vi "PromVIEW_GlobalOnCommand.vi"(10 "Command ID":string, 11 "Item Ref":T1) -> ()   [LabVIEW 2020]
uses:
  <resource>/Framework/Providers/API/ItemRef.ctl
panel:
  out "error out":errorcluster
  in  "error in":errorcluster
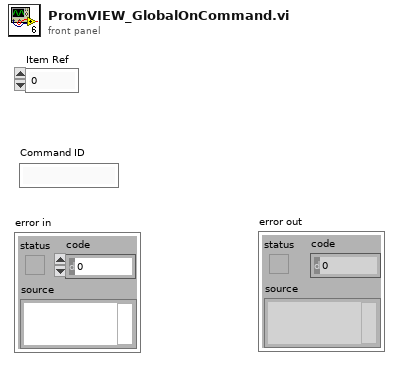
[diagram p1: front panel]
types:
  T1 = typedef "ItemRef.ctl" = u64
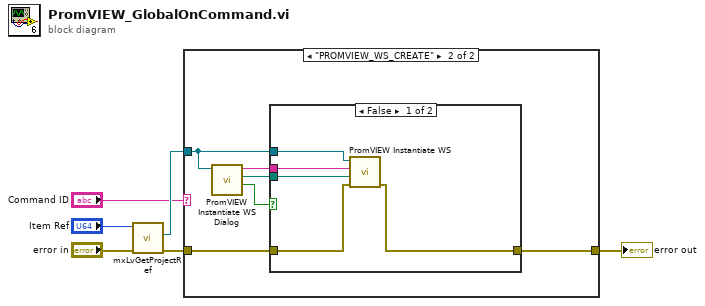
[diagram p0: block diagram]
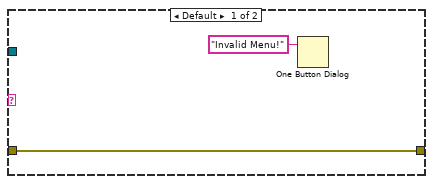
[diagram p2: hidden frame]
diagram:
  n1 = call <resource>:"mxLvGetProjectRef.vi"("error in"="error in", "Item"="Item Ref") -> ("error out"=w3:errorcluster, "Project Refnum"=w5:refnum<vi>)  [unwired: 7 in, 1 out]
  n2 = case shown="\"PROMVIEW_WS_CREATE\"" "Command ID" {
    tunnel: w5 -> [_ w14]
    tunnel: w3 -> [w8 w13]
    tunnel: [w8 w12] -> w2
    frame Default {
      n3 = One Button Dialog(message="Invalid Menu!") -> ()  [unwired: 1 in, 1 out]
    }
    frame "PROMVIEW_WS_CREATE" {
      n4 = call "PromVIEW Instantiate WS Dialog.vi"("Project Refnum"=w14) -> ("Cancelled"=w11:bool, "Web Resources Base Path out"=w9:path, "Web Service Name out"=w10:string)  [unwired: 8 in]
      n5 = case shown="False" w11 {
        tunnel: w14 -> [w19 _]
        tunnel: w10 -> [w18 _]
        tunnel: w9 -> [w17 _]
        tunnel: w13 -> [w16 w20]
        tunnel: [w15 w20] -> w12
        frame False {
          n6 = call "PromVIEW Instantiate WS.vi"("error in (no error)"=w16, "Web Resources Base Path"=w17, "Web Service Name"=w18, "Project Reference"=w19) -> ("Error Out"=w15:errorcluster)  [unwired: 7 in]
        }
        frame True {
        }
      }
    }
  }
  "error out" <- w2
